vi "Read Configuration.vi"(8 "error in (no error)":errorcluster, 11 "HECR in":refnum<class "PL SMC HECR.lvclass">) -> (0 "error out":errorcluster, 2 "configuration":T1={"control mode"=0, "Ttarget, °C"=25.0, "offset, °C"=0.0, "PID"={"PB range, °C"=6.0, "integral time, s"=18.0, "differential time, s"=0.0}, "heat output limit, %"=100.0, "cool output limit, %"=-100.0} {"control mode" items=["stop", "normal", "auto tuning", "learning", "external tune"]}, 3 "HECR out":refnum<class "PL SMC HECR.lvclass">)   [LabVIEW 2015, in "PL SMC HECR.lvclass"]
doc: "Reads device configuration."
uses:
  PL SMC HECR.lvclass
  <vilib>/plasmapper/PL Modbus Client/PL Modbus Client.lvclass
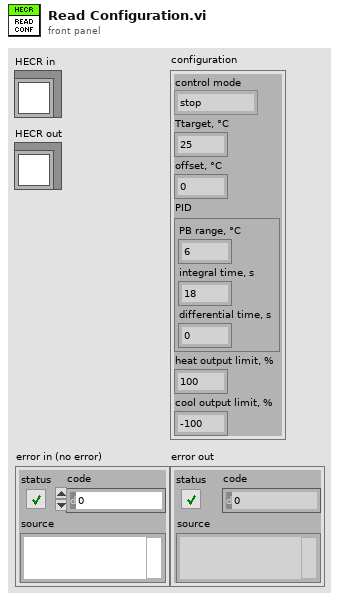
[diagram p1: front panel]
types:
  T1 = cluster{"control mode":u16, "Ttarget, °C":dbl, "offset, °C":dbl, "PID":cluster{"PB range, °C":dbl, "integral time, s":dbl, "differential time, s":dbl}, "heat output limit, %":dbl, "cool output limit, %":dbl}
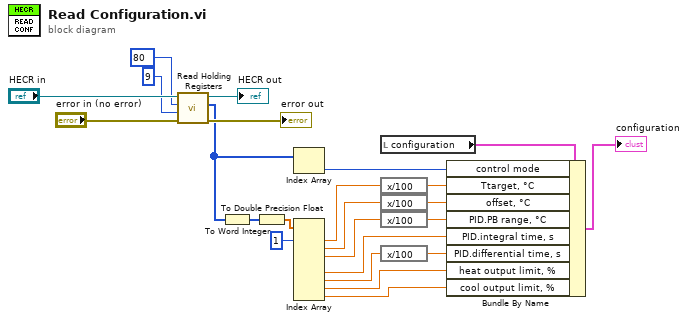
[diagram p0: block diagram]
diagram:
  n1 = call <vilib>:"Read Holding Registers.vi"("error in (no error)"="error in (no error)", "number of holding registers"=u16 9, "address"=u16 80, "MODBUS in"="HECR in") -> ("error out"=→"error out":errorcluster, "values"=w13:u16[], "MODBUS out"=→"HECR out":refnum<class "PL SMC HECR.lvclass">)  [unwired: 5 in]
  n2 = To Word Integer(number=w13) -> (16bit integer=w14:i16[])
  n3 = To Double Precision Float(number=w14) -> (double precision float=w16:dbl[])
  n4 = Index Array(array=w13) -> (element=w12:u16)  [unwired: 1 in]
  n5 = Index Array(array=w16, index #1=1 ("index")) -> (element #1=w11:dbl, element #2=w6:dbl, element #3=w5:dbl, element #5=w4:dbl, element #6=w3:dbl, element #7=w2:dbl, element #8=w1:dbl)  [unwired: 7 in, 1 out]
  n6 = local read "configuration"() -> (w18:T1)
  n7 = expression code="x/100"(w11) -> (w10:dbl)
  n8 = expression code="x/100"(w6) -> (w9:dbl)
  n9 = expression code="x/100"(w5) -> (w8:dbl)
  n10 = expression code="x/100"(w3) -> (w7:dbl)
  n11 = Bundle By Name(cluster=w18, "control mode"=w12, "Ttarget, °C"=w10, "offset, °C"=w9, "PID.PB range, °C"=w8, "PID.integral time, s"=w4, "PID.differential time, s"=w7, "heat output limit, %"=w2, "cool output limit, %"=w1) -> (→"configuration":T1)
